vi "Calculadora.vi"() -> ()   [LabVIEW 2019]
panel:
  out "Numeric":dbl
  in  "Boton /":bool
  in  "Boton *":bool
  in  "Boton-":bool
  in  "Boton =":bool
  in  "Boton 0":bool
  in  "Boton +":bool
  in  "Boton 9":bool
  in  "Boton 8":bool
  in  "Boton 7":bool
  in  "Boton 6":bool
  in  "Boton 5":bool
  in  "Boton 4":bool
  in  "Boton 3":bool
  in  "Boton 2":bool
  in  "Boton 1":bool
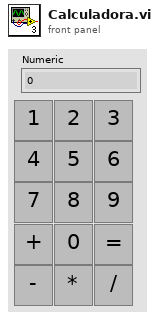
[diagram p1: front panel]
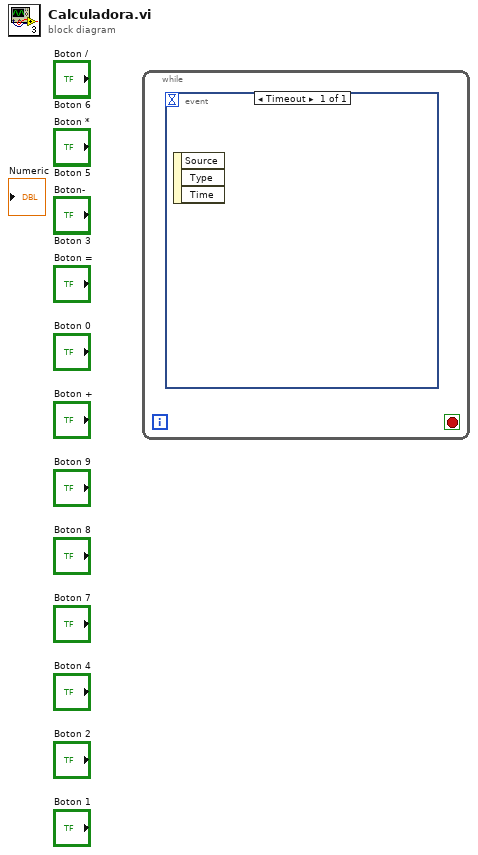
[diagram p0: block diagram]
diagram:
  n1 = while {
    stop <- _ stop-if-true
    n2 = event shown="[0] Timeout" {
      selector: _ -> [_]
      dyn-events: _ -> [_]
      timeout: _ -> [_]
      event Timeout {
        n3 = event-data() -> ()  [unwired: 1 in, 3 out]
      }
    }
  }
